vi "_DEPRICATED FRCts20_WebMethods_SetupDebug.vi"() -> ()   [LabVIEW 2014, in "FRCts20_WebMethods.lvlib"]
uses:
  FRCts20_WebMethods.lvlib
panel:
  out "Number of VIs fixed":i32
  out "Errors":errorcluster[](array[cluster])
  out "Number of Errors":i32
  out "Number of VIs found":i32
  in  "Setting":enum16{"Debug", "Deploy"}(ring)
  in  "VI Folder":path=path "D:/Parkway/Working Copy/Parkway/Web Methods/source/VI Source"
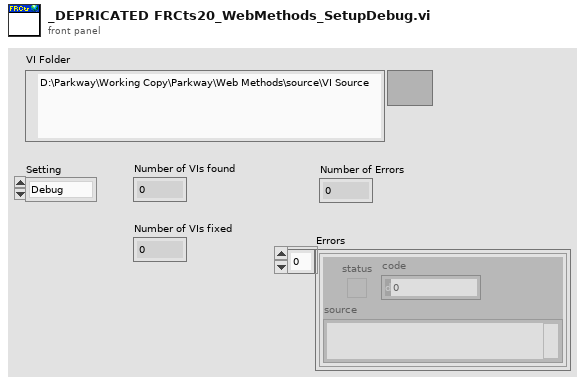
[diagram p1: front panel]
types:
  T1 = enum32{"Bad", "Idle", "Run top level", "Running"}
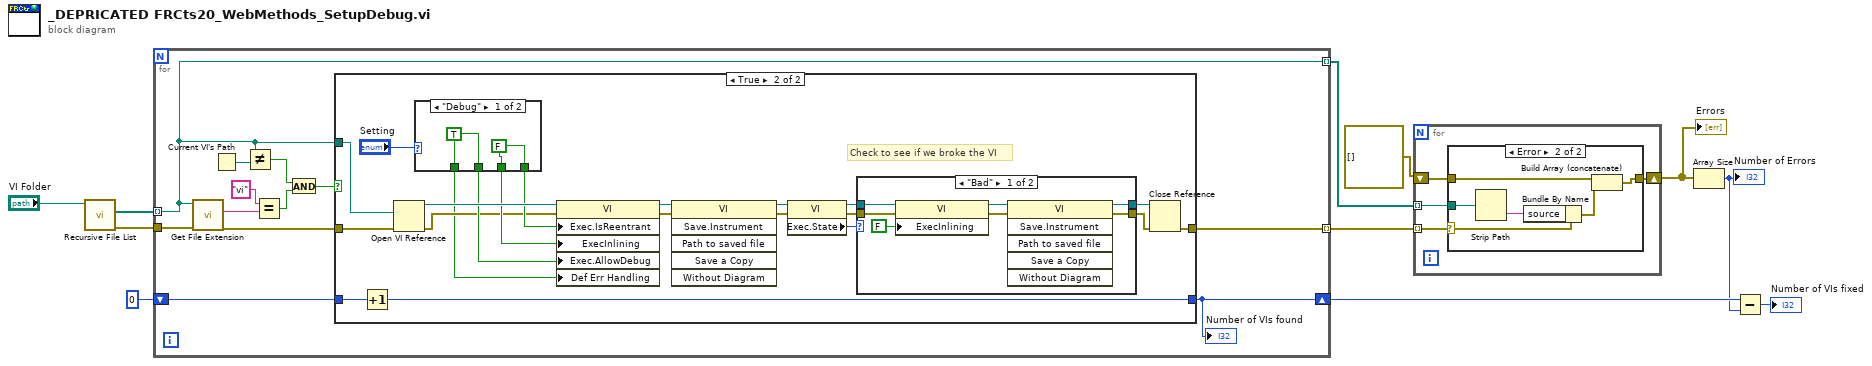
[diagram p0: block diagram]
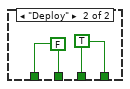
[diagram p5: hidden frame]
diagram:
  n1 = call <vilib>:"Recursive File List.vi"("Folder Path"="VI Folder") -> ("error out"=w10:errorcluster, "All Files in Dir"=w9:path[])  [unwired: 6 in, 3 out]
  n2 = for {
    tunnel: w9 -> [w18] mode=indexing
    tunnel: w10 -> [w23]
    shift-right: [w12] -> w3
    shift-left: 0 -> [w21]
    tunnel: [w20] -> w7 mode=indexing
    tunnel: [w18] -> w6 mode=indexing
    n3 = call <vilib>:"Get File Extension.vi"("error in (no error)"=w23, "file"=w18) -> ("error out"=w22:errorcluster, "lowercase file extension"=w17:string)  [unwired: 6 in, 2 out]
    n4 = Current VI's Path() -> (path=w19:path)
    n5 = Not Equal?(x=w18, y=w19) -> (x != y?=w14:bool)
    n6 = Equal?(x="vi" ("y"), y=w17) -> (x = y?=w15:bool)
    n7 = And(x=w14, y=w15) -> (x .and. y?=w13:bool)
    n8 = case shown="True" w13 {
      tunnel: w22 -> [w25 w46]
      tunnel: w18 -> [_ w45]
      tunnel: [w25 w38] -> w20
      tunnel: w21 -> [w24 w37]
      tunnel: [w24 w36] -> w12
      frame False {
      }
      frame True {
        # "Check to see if we broke the VI"
        n9 = Increment(x=w37) -> (x+1=w36:i32)
        n10 = Open VI Reference(vi path=w45, error in (no error)=w46) -> (vi reference=w43:refnum<vi>, error out=w39:errorcluster)  [unwired: 4 in]
        n11 = case shown="\"Debug\"" "Setting" {
          tunnel: [w57 w59] -> w42
          tunnel: [w57 w59] -> w41
          tunnel: [w56 w58] -> w40
          tunnel: [w56 w58] -> w35
          frame "Debug" {
            w57 = FALSE
            w56 = TRUE
          }
          frame "Deploy" {
            w58 = FALSE
            w59 = TRUE
          }
        }
        n12 = property class="VI"(reference=w43, error in=w39, "Exec.IsReentrant"=w42, "ExecInlining"=w41, "Exec.AllowDebug"=w40, "Def Err Handling"=w35) -> (reference out=w31:refnum<vi>, error out=w30:errorcluster)
        n13 = invoke class="VI" method="Save.Instrument"(reference=w31, error in=w30) -> (reference out=w28:refnum<vi>, error out=w29:errorcluster)  [unwired: 4 in, 4 out]
        n14 = property class="VI"(reference=w28, error in=w29) -> (reference out=w33:refnum<vi>, error out=w32:errorcluster, "Exec.State"=w34:T1)
        n15 = case shown="\"Bad\"" w34 {
          tunnel: w33 -> [w53 w55]
          tunnel: w32 -> [w52 w54]
          tunnel: [w47 w54] -> w26
          tunnel: [w48 w55] -> w27
          frame "Bad" {
            n16 = property class="VI"(reference=w53, error in=w52, "ExecInlining"=FALSE ("Execution:Inline SubVI")) -> (reference out=w50:refnum<vi>, error out=w49:errorcluster)
            n17 = invoke class="VI" method="Save.Instrument"(reference=w50, error in=w49) -> (reference out=w48:refnum<vi>, error out=w47:errorcluster)  [unwired: 4 in, 4 out]
          }
          frame Default {
          }
        }
        n18 = Close Reference(reference=w27, error in (no error)=w26) -> (error out=w38:errorcluster)
      }
    }
    "Number of VIs found" <- w12
  }
  n19 = for {
    tunnel: w7 -> [w63] mode=indexing
    tunnel: w6 -> [w61] mode=indexing
    shift-right: [w60] -> w4
    shift-left: errorcluster[] [] -> [w62]
    n20 = case shown="Error" w63 {
      selector: w63 -> [_ w69]
      tunnel: w62 -> [w64 w70]
      tunnel: w61 -> [_ w66]
      tunnel: [w64 w67] -> w60
      frame No Error {
      }
      frame Error {
        n21 = Strip Path(path=w66) -> (name=w65:string)  [unwired: 1 out]
        n22 = Bundle By Name(cluster=w69, "source"=w65) -> (w68:errorcluster)
        n23 = Build Array (concatenate)(w70, w68) -> (w67:errorcluster[])
      }
    }
  }
  "Errors" <- w4
  n24 = Array Size(array=w4) -> (size(s)=w2:i32)
  "Number of Errors" <- w2
  n25 = Subtract(x=w3, y=w2) -> (x-y=→"Number of VIs fixed":i32)
